vi "IsRefnum.vi"(8 "error in":errorcluster, 11 "StepRun in":refnum<class "StepRun.lvclass">) -> (0 "error out":errorcluster, 2 "IsRefnum":bool, 3 "StepRun out":refnum<class "StepRun.lvclass">)   [LabVIEW 2021, in "ProligentXMLGenerator.lvlib" / "StepRun.lvclass"]
doc: "Returns TRUE if the passed object is valid."
uses:
  StepRun.lvclass
  StepRun.lvclass/StepRun.ctl
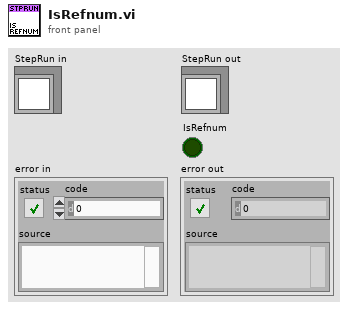
[diagram p1: front panel]
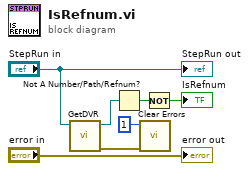
[diagram p0: block diagram]
diagram:
  n1 = call "GetDVR.vi"("StepRun"="StepRun in") -> ("error out"=w1:errorcluster, "DVRReference"=w3:refnum<data-value>)  [unwired: 9 in]
  n2 = Not A Number/Path/Refnum?(number/path/refnum=w3) -> (NaN/Path/Refnum?=w5:bool)
  n3 = call <vilib>:"Clear Errors.vi"("error in (no error)"=w1, "specific error code to clear (0: all)"=1) -> ()  [unwired: 4 in, 2 out]
  n4 = Not(x=w5) -> (.not. x?=→"IsRefnum":bool)
  "error out" <- "error in"
  "StepRun out" <- "StepRun in"
